vi "time multiply_v2.vi"() -> ()   [LabVIEW 2020]
uses:
  <vilib>/Analysis/Matrix/Numeric/Conversions/Array To Matrix - RA.vi
  <vilib>/Analysis/Matrix/Numeric/Conversions/Array To Matrix - RA2.vi
  <vilib>/Analysis/Matrix/Numeric/Multiply/Multiply - RM,RM.vi
  <vilib>/Analysis/Matrix/NI_Matrix.lvlib
panel:
  out "average time":dbl
  in  "vector size":i32=20
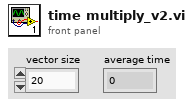
[diagram p1: front panel]
types:
  T1 = typedef "NI_Matrix.lvlib/RealMatrix.ctl" = dbl[][]
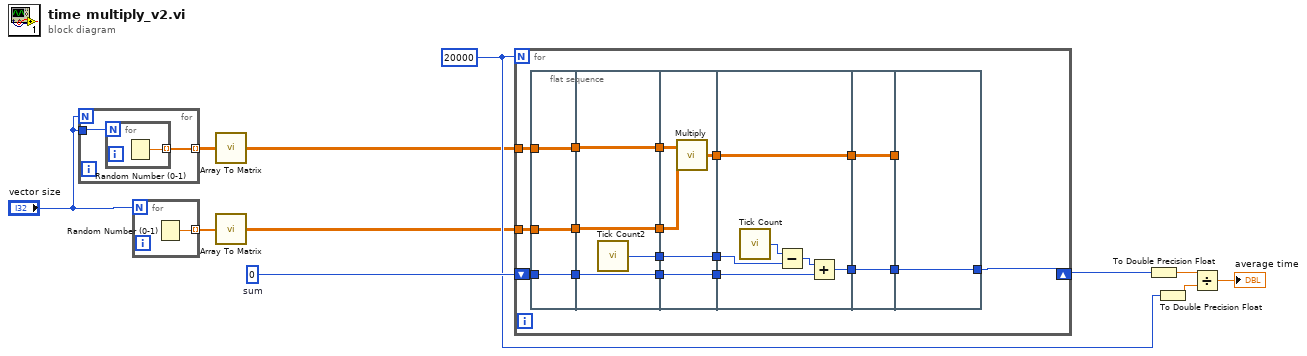
[diagram p0: block diagram]
diagram:
  w11 = u32 0  # sum
  w8 = 20000
  n1 = for {
    N: "vector size" -> [_]
    tunnel: [w13] -> w4 mode=indexing
    tunnel: "vector size" -> [w12]
    n2 = for {
      N: w12 -> [_]
      tunnel: [w14] -> w13 mode=indexing
      n3 = Random Number (0-1)() -> (number: 0 to 1=w14:dbl)
    }
  }
  n4 = for {
    N: "vector size" -> [_]
    tunnel: [w15] -> w3 mode=indexing
    n5 = Random Number (0-1)() -> (number: 0 to 1=w15:dbl)
  }
  n6 = call-poly <vilib>:"Array To Matrix.vi"("Real 2D Array"=w4) -> ("Real Matrix"=w2:T1)
  n7 = call-poly <vilib>:"Array To Matrix.vi"("Real 1D Array"=w3) -> ("Real Matrix (Column Vector)"=w1:T1)
  n8 = for {
    N: w8 -> [_]
    shift-right: [w22] -> w10
    shift-left: w11 -> [w23]
    tunnel: w2 -> [w21]
    tunnel: w1 -> [w20]
    n9 = flat-sequence {
      tunnel: [w34] -> w33
      tunnel: [w35] -> w27
      tunnel: [w36] -> w24
      tunnel: w23 -> [w36]
      tunnel: w21 -> [w35]
      tunnel: w20 -> [w34]
      tunnel: w33 -> [w40]
      tunnel: [w40] -> w32
      tunnel: [w39] -> w31
      tunnel: [w38] -> w28
      tunnel: w27 -> [w38]
      tunnel: [w37] -> w25
      tunnel: w24 -> [w37]
      tunnel: w32 -> [w43]
      tunnel: w31 -> [w45]
      tunnel: [w45] -> w30
      tunnel: [w42] -> w29
      tunnel: w28 -> [w44]
      tunnel: [w41] -> w26
      tunnel: w25 -> [w41]
      tunnel: w29 -> [w49]
      tunnel: w30 -> [w50]
      tunnel: [w49] -> w19
      tunnel: w26 -> [w47]
      tunnel: [w46] -> w17
      tunnel: w19 -> [w53]
      tunnel: [w53] -> w18
      tunnel: w17 -> [w52]
      tunnel: [w52] -> w16
      tunnel: w18 -> [_]
      tunnel: [w54] -> w22
      tunnel: w16 -> [w54]
      frame #0 {
      }
      frame #1 {
        n10 = call "Tick Count2"() -> ("Tick Count(uSec)"=w39:u32)
      }
      frame #2 {
        n11 = call-poly <vilib>:"Multiply.vi"("Real Matrix B"=w43, "Real Matrix A"=w44) -> ("A * B"=w42:T1)
      }
      frame #3 {
        n12 = call "Tick Count"() -> ("Tick Count(uSec)"=w51:u32)
        n13 = Subtract(x=w51, y=w50) -> (x-y=w48:u32)
        n14 = Add(x=w48, y=w47) -> (x+y=w46:u32)
      }
      frame #4 {
      }
      frame #5 {
      }
    }
  }
  n15 = To Double Precision Float(number=w10) -> (double precision float=w7:dbl)
  n16 = To Double Precision Float(number=w8) -> (double precision float=w9:dbl)
  n17 = Divide(x=w7, y=w9) -> (x/y=→"average time":dbl)
